vi "Splash Screen.vi"() -> ()   [LabVIEW 2023, in "GUI.lvlib" / "Vitesco Launcher.lvlib"]
doc: "This is the top-level VI of this application. When it runs, it behaves like the splash screen many applications use to keep the user occupied while the application loads into memory. This application is quite small, so there is little overhead, which would make the splash screen just flash for a moment. Because that flash is distracting, there is a three-second delay inserted into this VI so that it stays up for a little bit. \n\nThis VI uses a delay-loaded subVI call to load the rest of the application. This trick ensures that the splash screen can load instantly regardless of how large the rest of the VI hierarchy gets, and the loading of the rest of the VIs becomes one step in the load process."
uses:
  Vitesco Launcher.lvlib
  Actor/Main/Main/Main.lvclass
  NationalInstruments.TestStand.Interop.API
  <vilib>/ActorFramework/Actor/Actor.lvclass
panel:
  out "version":string
  in  "error in (no error)":errorcluster
  # "eDCU \nLIFE TIME TESTER"
  # "Initializing...."
  # "Designed and Developed by"
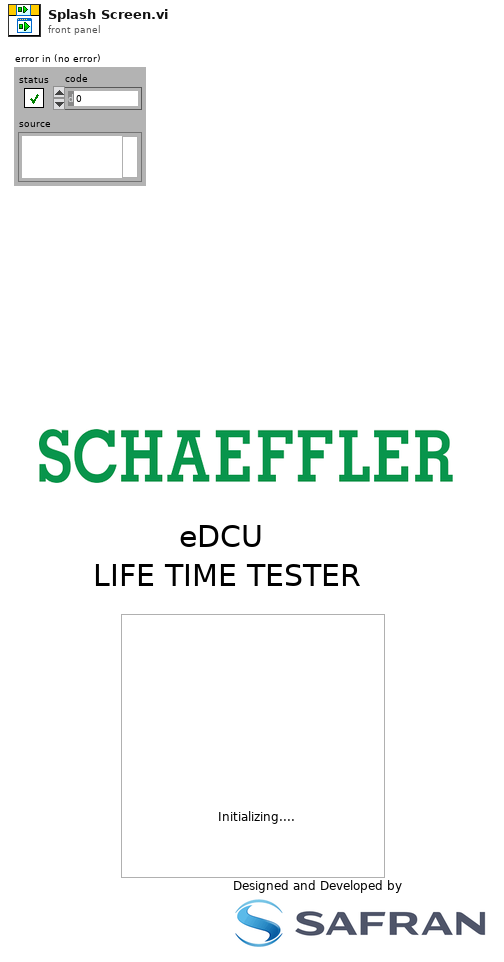
[diagram p1: front panel]
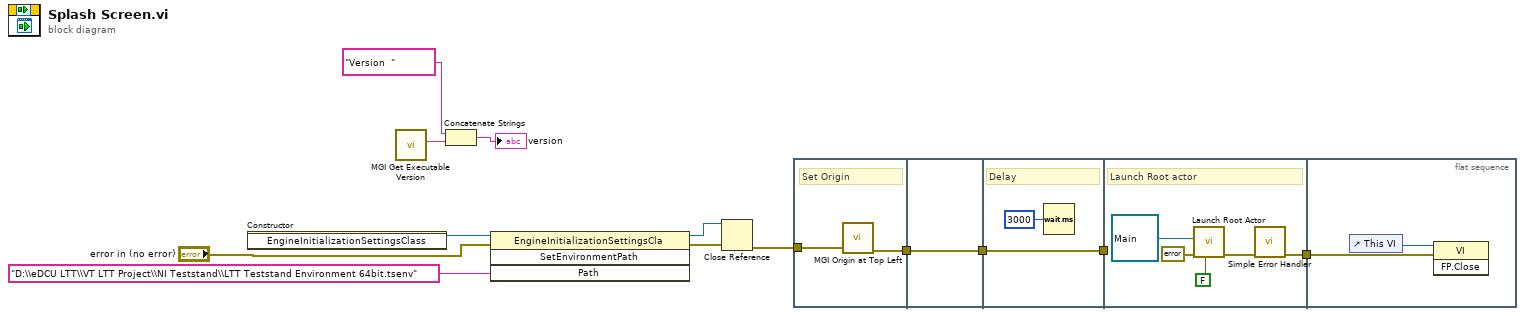
[diagram p0: block diagram]
diagram:
  n1 = constructor class="EngineInitializationSettingsCla"() -> (reference out=w11:refnum<k24>)  [unwired: 3 in, 2 out]
  n2 = call <userlib>:"MGI Get Executable Version.vi"() -> ("Version"=w1:string)  [unwired: 7 in]
  n3 = Concatenate Strings("Version  " ("string"), w1) -> (→"version":string)
  n4 = invoke class="EngineInitializationSettingsCla" method="SetEnvironmentPath"(reference=w11, error in="error in (no error)", "Path"="D:\\eDCU LTT\\VT LTT Project\\NI Teststand\\LTT Teststand Environment 64bit.tsenv") -> (reference out=w9:refnum<k24>, error out=w10:errorcluster)  [unwired: 1 in, 2 out]
  n5 = Close Reference(reference=w9, error in (no error)=w10) -> (error out=w6:errorcluster)
  n6 = flat-sequence {
    tunnel: w6 -> [w14]
    tunnel: [w15] -> w12
    tunnel: w12 -> [w16]
    tunnel: [w16] -> w5
    tunnel: w5 -> [w17]
    tunnel: [w17] -> w4
    tunnel: [w23] -> w13
    tunnel: w4 -> [_]
    tunnel: w13 -> [w25]
    frame #0 {
      # "Set Origin"
      n7 = call <userlib>:"MGI Origin at Top Left.vi"("Error In"=w14) -> ("Error Out"=w15:errorcluster)  [unwired: 8 in, 1 out]
    }
    frame #1 {
    }
    frame #2 {
      # "Delay"
      n8 = Wait (ms)(milliseconds to wait=u32 3000) -> ()  [unwired: 1 out]
    }
    frame #3 {
      # "Launch Root actor"
      n9 = call <vilib>:"Launch Root Actor.vi"("Open Actor Core front panel? (F)"=FALSE, "error in (no error)"=errorcluster {"status"=FALSE, "code"=0, "source"=""}, "Actor"=refnum<class "Main.lvclass"> refnum ("GUI.lvlib:Main.lvlib:Main.lvclass")) -> ("error out"=w22:errorcluster)  [unwired: 7 in, 1 out]
      n10 = call <vilib>:"Simple Error Handler.vi"("error in (no error)"=w22) -> ("error out"=w23:errorcluster)  [unwired: 4 in, 4 out]
    }
    frame #4 {
      n11 = control-ref of="This VI"() -> (w24:refnum<vi>)
      n12 = invoke class="VI" method="FP.Close"(reference=w24, error in=w25) -> ()  [unwired: 1 in, 3 out]
    }
  }
